vi "Log Message.vi"(8 "error in (no error)":errorcluster, 9 "String":string, 10 "Source Name":string, 11 "cRIO-CO2 in":refnum<class "cRIO-CO2.lvclass">) -> (0 "error out":errorcluster, 3 "cRIO-CO2 out":refnum<class "cRIO-CO2.lvclass">)   [LabVIEW 2015, in "cRIO-Carbondioxide.lvlib" / "cRIO-CO2.lvlib" / "cRIO-CO2.lvclass"]
uses:
  cRIO-CO2.lvclass
  cRIO-CO2.lvclass/cRIO-CO2.ctl
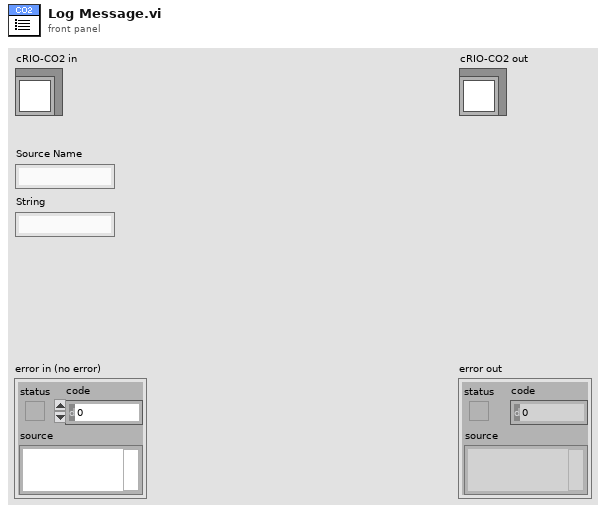
[diagram p1: front panel]
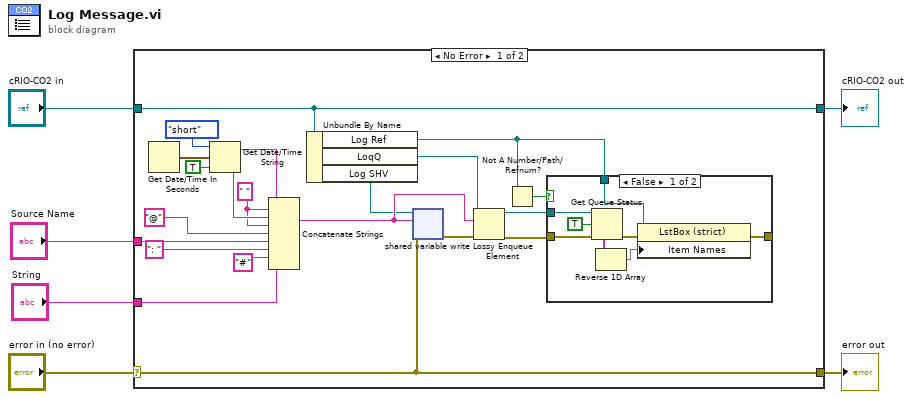
[diagram p0: block diagram]
diagram:
  n1 = case shown="No Error" "error in (no error)" {
    selector: "error in (no error)" -> [w11 w38]
    tunnel: [w11 w38] -> w5
    tunnel: [w27 w37] -> w3
    tunnel: "cRIO-CO2 in" -> [w27 w37]
    tunnel: "Source Name" -> [w25 _]
    tunnel: "String" -> [w23 _]
    frame No Error {
      w16 = " "
      n2 = Get Date/Time In Seconds() -> (seconds since 1Jan1904=w22:timestamp)
      n3 = Get Date/Time String(date format (0)=enum16{"short", "long", "abbreviated"}."short", seconds (now)=w22, want seconds? (F)=TRUE) -> (date string=w18:string, time string=w17:string)
      n4 = Concatenate Strings(w18, w16, w17, w16, "@" ("string"), w25, ": " ("string"), "#" ("string"), w23) -> (w9:string)
      n5 = Unbundle By Name(w27) -> ("Log Ref"=w13:refnum<vi>, "LoqQ"=w15:refnum<queue>, "Log SHV"=w8:refnum<k21>)
      n6 = shared-variable-write(w8, w11, w9) -> (w14:errorcluster)  [unwired: 1 out]
      n7 = Lossy Enqueue Element(queue=w15, element=w9, error in (no error)=w14) -> (queue out=w26:refnum<queue>, error out=w10:errorcluster)  [unwired: 2 out]
      n8 = Not A Number/Path/Refnum?(number/path/refnum=w13) -> (NaN/Path/Refnum?=w12:bool)
      n9 = case shown="False" w12 {
        tunnel: w13 -> [w35 _]
        tunnel: w26 -> [w34 _]
        tunnel: w10 -> [w31 w36]
        tunnel: [w28 w36] -> _
        frame False {
          n10 = Get Queue Status(queue=w34, return elements? (F)=TRUE, error in (no error)=w31) -> (error out=w29:errorcluster, elements=w32:string[])  [unwired: 6 out]
          n11 = Reverse 1D Array(array=w32) -> (reversed array=w30:string[])
          n12 = property class="LstBox (strict)"(reference=w35, error in=w29, "Item Names"=w30) -> (error out=w28:errorcluster)  [unwired: 1 out]
        }
        frame True {
        }
      }
    }
    frame Error {
    }
  }
  "error out" <- w5
  "cRIO-CO2 out" <- w3
